vi "Rework_Calculate-1.vi"(9 "Rework站号":string, 10 "当前站号":string) -> (1 "Data":string[](array[string]), 2 "Rework_List":string[](array[string]), 3 "跨站":bool)   [LabVIEW 2018]
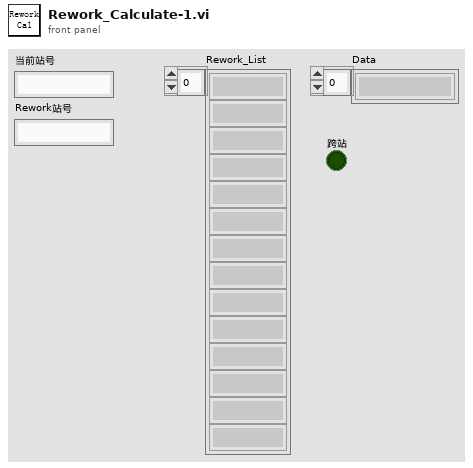
[diagram p1: front panel]
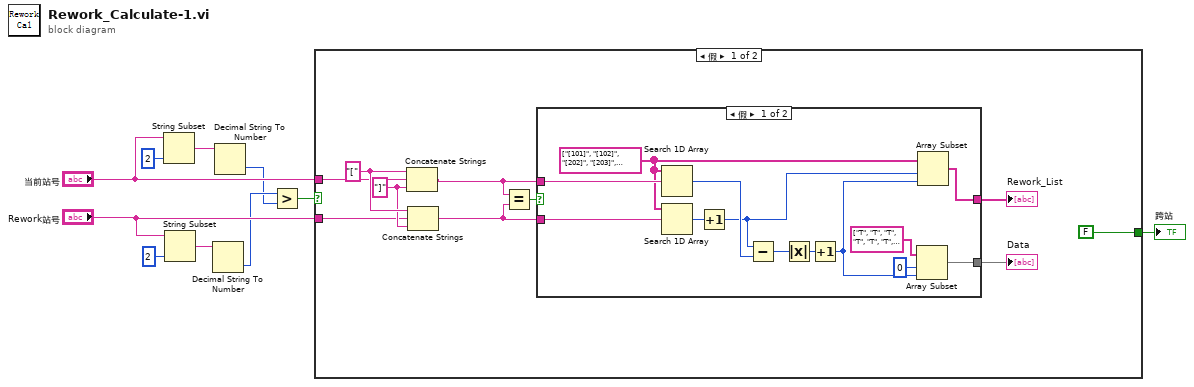
[diagram p0: block diagram]
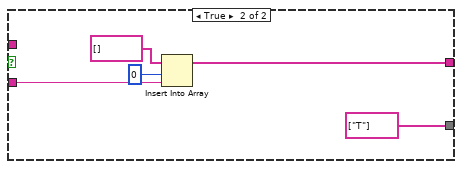
[diagram p2: hidden frame]
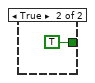
[diagram p3: hidden frame]
diagram:
  n1 = String Subset(string="当前站号", length (rest)=2 ("长度（剩余）")) -> (substring=w5:string)  [unwired: 1 in]
  n2 = String Subset(string="Rework站号", length (rest)=2 ("长度（剩余）")) -> (substring=w6:string)  [unwired: 1 in]
  n3 = Decimal String To Number(string=w6) -> (number=w4:i32)  [unwired: 2 in, 1 out]
  n4 = Decimal String To Number(string=w5) -> (number=w3:i32)  [unwired: 2 in, 1 out]
  n5 = Greater?(x=w4, y=w3) -> (0:w2:bool)
  n6 = case shown="假" w2 {
    tunnel: "当前站号" -> [w13 _]
    tunnel: "Rework站号" -> [w12 _]
    tunnel: [FALSE TRUE] -> w1
    frame False {
      w14 = "]" ("字符串")
      w15 = "[" ("字符串")
      n7 = Concatenate Strings(w15, w13, w14) -> (w17:string)
      n8 = Concatenate Strings(w15, w12, w14) -> (w16:string)
      n9 = Equal?(x=w17, y=w16) -> (x = y?=w20:bool)
      n10 = case shown="假" w20 {
        tunnel: w16 -> [w32 w38]
        tunnel: [w29 w35] -> w19
        tunnel: [w22 string[] ["T"]] -> w18
        tunnel: w17 -> [w33 _]
        frame False {
          w21 = string[] ["[101]", "[102]", "[202]", "[203]", "[301]", "[302]", "[401]", "[403]", "[502]", "[503]", "[601]", "[602]", "[70]"]
          n11 = Search 1D Array(1D array=w21, element=w33) -> (index of element=w31:i32)  [unwired: 1 in]
          n12 = Search 1D Array(1D array=w21, element=w32) -> (index of element=w25:i32)  [unwired: 1 in]
          n13 = Increment(x=w25) -> (x+1=w24:i32)
          n14 = Subtract(x=w24, y=w31) -> (x-y=w30:i32)
          n15 = Absolute Value(x=w30) -> (abs(x)=w27:i32)
          n16 = Increment(x=w27) -> (x+1=w26:i32)
          n17 = Array Subset(array=string[] ["T", "T", "T", "T", "T", "T", "T", "T", "T", "T", "T", "T", "T", "T", "T", "T", "T", "T", "T", "T", "T"], index=0 ("索引"), length=w26) -> (w22:string[])
          n18 = Array Subset(array=w21, index=w24, length=w26) -> (w29:string[])
        }
        frame True {
          n19 = Insert Into Array(array=string[] [] ("数组"), index=0 ("索引"), new element=w38) -> (w35:string[])
        }
      }
      "Rework_List" <- w19
      "Data" <- w18
    }
    frame True {
    }
  }
  "跨站" <- w1
